vi "is_valid.vi"(11 "Headers in":refnum<class "Headers.lvclass">) -> (2 "valid-ref?":bool)   [LabVIEW 2020, in "reqwest.lvlib" / "Headers.lvclass"]
uses:
  Headers.lvclass
  Headers.lvclass/Headers.ctl
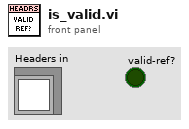
[diagram p1: front panel]
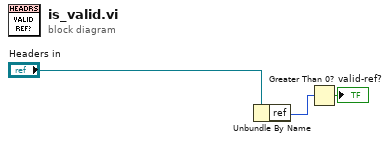
[diagram p0: block diagram]
diagram:
  n1 = Unbundle By Name("Headers in") -> ("ref"=w2:u64)
  n2 = Greater Than 0?(x=w2) -> (x > 0?=→"valid-ref?":bool)
